vi "系统设置.vi"() -> ()   [LabVIEW 2016]
uses:
  <vilib>/Utility/miscctls.llb/LVPointTypeDef.ctl
  <vilib>/Utility/config.llb/Read Key (I32).vi
  <vilib>/Utility/config.llb/Read Key (Boolean).vi
  PLC/PLC.lvlib
  <vilib>/ptbypt/NI_PtbyPt.lvlib
  <vilib>/Utility/config.llb/NI_LVConfig.lvlib
panel:
  out "周期参数":T1
  in  "周期设置":bool
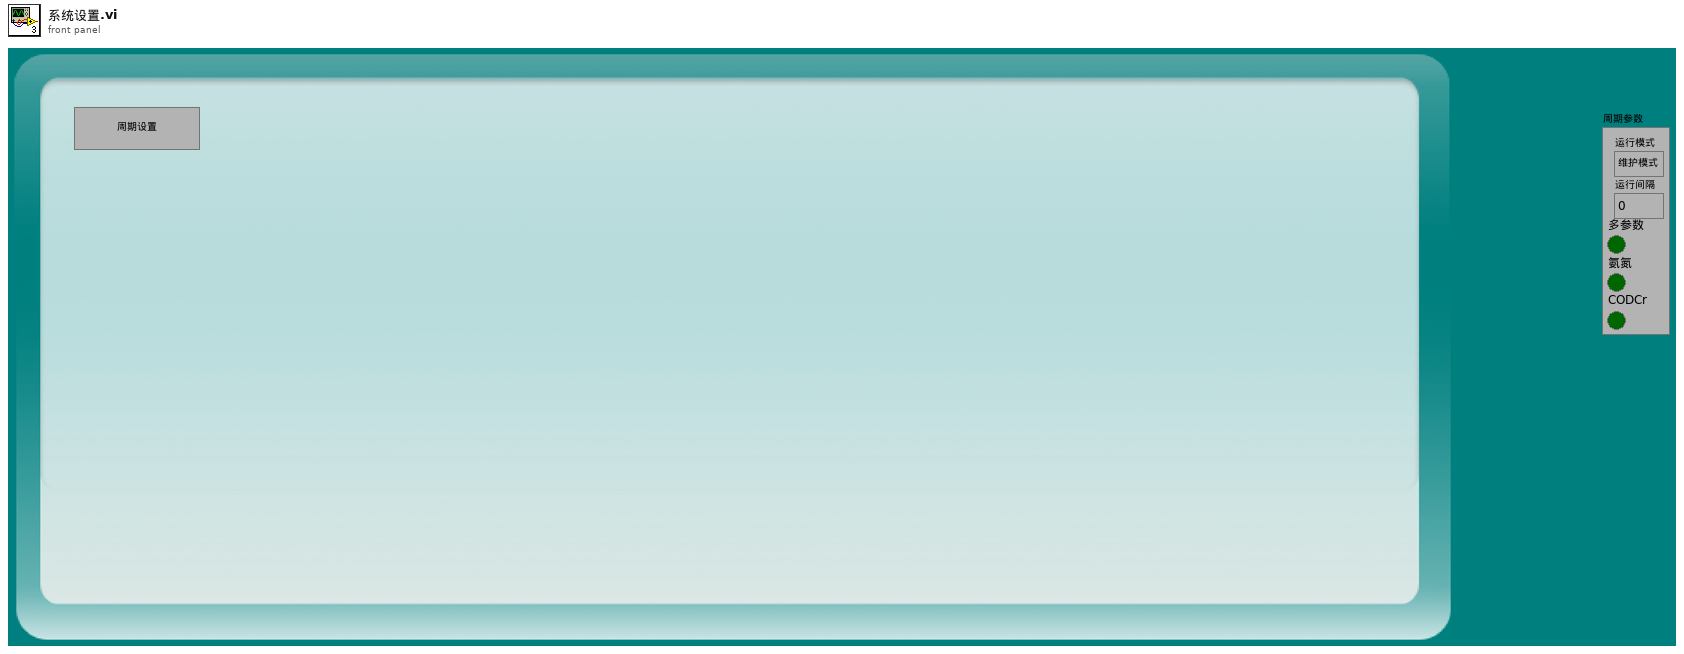
[diagram p1: front panel]
types:
  T1 = cluster{"运行模式":enum16{"维护模式", "常规模式", "应急模式", "质控模式"}, "运行间隔":i16, "多参数":bool, "氨氮":bool, "CODCr":bool}
  T2 = typedef "LVPointTypeDef.ctl" = cluster{"Horizontal":i16, "Vertical":i16}
  T3 = cluster{"CODCr":cluster{"启动测量模式":cluster{"测量模式":enum16{"水样测量", "标样核查", "零点核查", "加标回收", "平行样", "校零", "校标"}}, "确定按钮":bool}, "参数启用":cluster{"多参数":bool, "CODMn":bool, "总磷总氮":bool, "氨氮":bool, "CODcr":bool}}
  T4 = enum16{"水样测量", "标样核查", "零点核查", "加标回收", "平行样", "校零", "校标"}
  T5 = typedef "LVDateTimeRec.ctl" = cluster{"秒数的小数部分":dbl, "秒":i32, "分":i32, "时":i32, "日":i32, "月":i32, "年":i32, "天数（周）":i32, "天数（年）":i32, "DST":i32}
  T6 = typedef "NI_LVConfig.lvlib/Config Data RefNum.ctl" = refnum<k1>
  T7 = cluster{"value":i32, "value":i32, "value":bool, "value":bool, "value":bool}
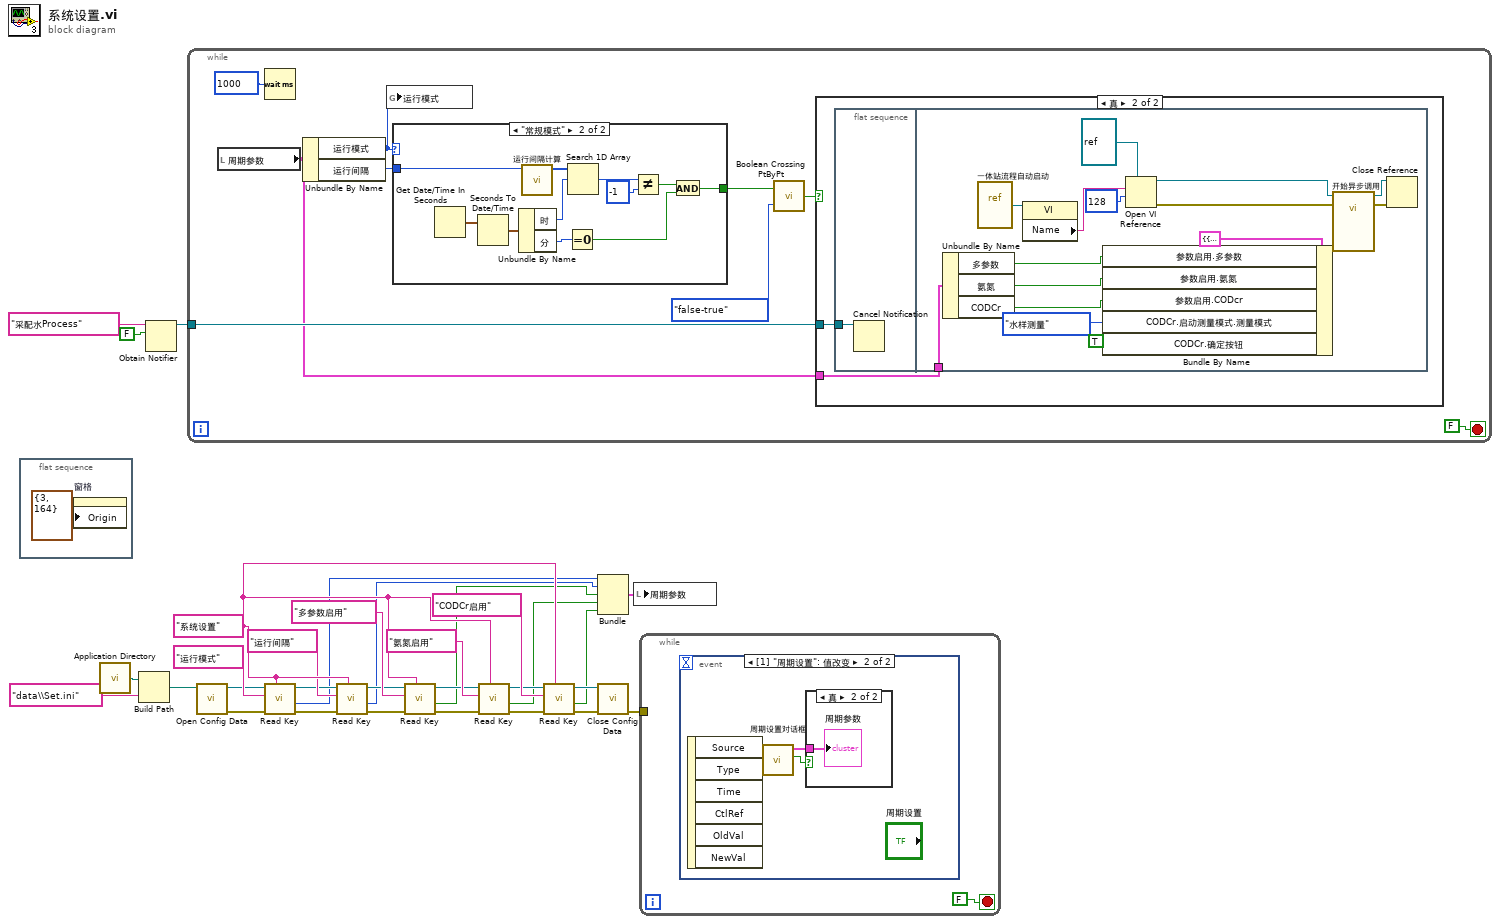
[diagram p0: block diagram]
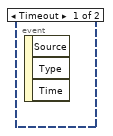
[diagram p4: hidden frame]
diagram:
  w25 = "系统设置" ("section")
  n1 = flat-sequence {
    frame #0 {
      n2 = property on="窗格" class="Pane"("Origin"=T2 {"Horizontal"=3, "Vertical"=164} ("原点")) -> ()  [unwired: 2 in, 2 out]
    }
  }
  n3 = call <vilib>:"Application Directory.vi"() -> ("Application Directory"=w10:path)
  n4 = Build Path(base path=w10, name or relative path="data\\Set.ini" ("名称或相对路径")) -> (appended path=w12:path)
  n5 = Obtain Notifier(name (unnamed)="采配水Process" ("名称（未命名）"), notification data type=FALSE) -> (notifier out=w29:refnum<notifier>)  [unwired: 2 in, 2 out]
  n6 = while {
    tunnel: w29 -> [w39]
    stop <- FALSE stop-if-true
    n7 = local read "周期参数"() -> (w33:T1)
    n8 = Wait (ms)(milliseconds to wait=u32 1000 ("等待时间（毫秒）")) -> ()  [unwired: 1 out]
    n9 = Unbundle By Name(w33) -> ("运行模式"=w35:enum16{"维护模式", "常规模式", "应急模式", "质控模式"}, "运行间隔"=w34:i16)
    n10 = global write "系统变量.vi" "运行模式"(w35) -> ()
    n11 = case shown="\"常规模式\"" w35 {
      tunnel: [_ w62] -> w38
      tunnel: w34 -> [_ w61]
      frame "维护模式", Default {
      }
      frame "常规模式" {
        n12 = Get Date/Time In Seconds() -> (seconds since 1Jan1904=w71:timestamp)
        n13 = Seconds To Date/Time(time stamp (now)=w71) -> (date time rec=w70:T5)  [unwired: 1 in]
        n14 = Unbundle By Name(w70) -> ("时"=w67:i32, "分"=w69:i32)
        n15 = call "运行间隔计算.vi"("运行周期"=w61) -> ("数组"=w68:i32[])  [unwired: 10 in]
        n16 = Equal To 0?(x=w69) -> (x = 0?=w63:bool)
        n17 = Search 1D Array(1D array=w68, element=w67) -> (index of element=w66:i32)  [unwired: 1 in]
        n18 = Not Equal?(x=w66, y=-1) -> (x != y?=w64:bool)
        n19 = And(x=w64, y=w63) -> (x .and. y?=w62:bool)
      }
    }
    n20 = call <vilib>:"Boolean Crossing PtByPt.vi"("direction"=enum16{"either", "false-true", "true-false"}."false-true", "input"=w38) -> ("crossing"=w36:bool)  [unwired: 1 in]
    n21 = case shown="真" w36 {
      tunnel: w39 -> [_ w43]
      tunnel: w33 -> [_ w42]
      frame False {
      }
      frame True {
        n22 = flat-sequence {
          tunnel: w43 -> [w44]
          tunnel: w42 -> [w51]
          frame #0 {
            n23 = Cancel Notification(0:w44) -> ()  [unwired: 1 in, 3 out]
          }
          frame #1 {
            n24 = Unbundle By Name(w51) -> ("多参数"=w50:bool, "氨氮"=w49:bool, "CODCr"=w48:bool)
            n25 = vi-ref "一体站流程自动启动.vi"() -> (w60:refnum<vi>)
            n26 = property class="VI"(reference=w60) -> ("Name"=w59:string)  [unwired: 1 in, 2 out]
            n27 = Bundle By Name(cluster=T3 {"CODCr"={"启动测量模式"={"测量模式"=enum."水样测量"}, "确定按钮"=TRUE}, "参数启用"={"多参数"=FALSE, "CODMn"=FALSE, "总磷总氮"=FALSE, "氨氮"=FALSE, "CODcr"=FALSE}} ("参数"), "参数启用.多参数"=w50, "参数启用.氨氮"=w49, "参数启用.CODcr"=w48, "CODCr.启动测量模式.测量模式"=T4."水样测量" ("CODMn.启动测量模式.测量模式"), "CODCr.确定按钮"=TRUE ("CODMn.确定按钮")) -> (w45:T3)
            n28 = Open VI Reference(type specifier VI Refnum (for type only)=refnum<vi> refnum ("类型说明符VI引用句柄（仅用于类型）"), vi path=w59, options=128 ("选项")) -> (vi reference=w57:refnum<vi>, error out=w55:errorcluster)  [unwired: 3 in]
            n29 = call-by-ref "开始异步调用"(reference=w57, error in=w55, "参数"=w45) -> (reference out=w56:refnum<vi>, error out=w54:errorcluster)  [unwired: 11 in]
            n30 = Close Reference(reference=w56, error in (no error)=w54) -> ()  [unwired: 1 out]
          }
        }
      }
    }
  }
  n31 = call <vilib>:"Open Config Data.vi"("configuration file path"=w12) -> ("error out"=w9:errorcluster, "refnum"=w8:T6)  [unwired: 8 in, 1 out]
  n32 = call-poly <vilib>:"Read Key.vi"("section"=w25, "error in (no error)"=w9, "key"="运行模式" ("section"), "refnum"=w8) -> ("error out"=w14:errorcluster, "value"=w6:i32, "refnum out"=w13:T6)  [unwired: 4 in, 1 out]
  n33 = call-poly <vilib>:"Read Key.vi"("section"=w25, "error in (no error)"=w14, "key"="运行间隔" ("section"), "refnum"=w13) -> ("error out"=w21:errorcluster, "value"=w5:i32, "refnum out"=w19:T6)  [unwired: 4 in, 1 out]
  n34 = call-poly <vilib>:"Read Key.vi"("section"=w25, "error in (no error)"=w21, "key"="多参数启用" ("section"), "refnum"=w19) -> ("error out"=w17:errorcluster, "value"=w4:bool, "refnum out"=w18:T6)  [unwired: 4 in, 1 out]
  n35 = call-poly <vilib>:"Read Key.vi"("section"=w25, "error in (no error)"=w17, "key"="氨氮启用" ("section"), "refnum"=w18) -> ("error out"=w22:errorcluster, "value"=w3:bool, "refnum out"=w20:T6)  [unwired: 4 in, 1 out]
  n36 = call-poly <vilib>:"Read Key.vi"("section"=w25, "error in (no error)"=w22, "key"="CODCr启用" ("section"), "refnum"=w20) -> ("error out"=w23:errorcluster, "value"=w2:bool, "refnum out"=w24:T6)  [unwired: 4 in, 1 out]
  n37 = Bundle("value"=w6, "value"=w5, "value"=w4, "value"=w3, "value"=w2) -> (w1:T7)  [unwired: 1 in]
  n38 = call <vilib>:"Close Config Data.vi"("error in (no error)"=w23, "refnum"=w24) -> ("error out"=w7:errorcluster)  [unwired: 8 in, 1 out]
  n39 = local write "周期参数"(w1) -> ()
  n40 = while {
    tunnel: w7 -> [_]
    stop <- FALSE stop-if-true
    n41 = event shown="[1] \"周期设置\": 值改变" {
      selector: _ -> [_ _]
      dyn-events: _ -> [_ _]
      timeout: _ -> [_ _]
      event Timeout {
        n42 = event-data() -> ()  [unwired: 1 in, 3 out]
      }
      event "周期设置": Value Change {
        n43 = event-data() -> ()  [unwired: 1 in, 6 out]
        n44 = call "周期设置对话框.vi"() -> ("确定"=w74:bool, "输出簇"=w73:T1)  [unwired: 10 in]
        n45 = case shown="真" w74 {
          tunnel: w73 -> [_ w75]
          frame False {
          }
          frame True {
            "周期参数" <- w75
          }
        }
      }
    }
  }
